vi "Create Log Sink Reference.vi"(8 "Error In":errorcluster, 11 "Log Sink":refnum<class "Log Sink.lvclass">) -> (0 "Error Out":errorcluster, 3 "Log Sink Reference":refnum<data-value>)   [LabVIEW 2016, in "Stream Log.lvlib" / "Log Sink.lvclass"]
doc: "--\nCopyright © 2017 Composed SystemsI All rights reserved.\n\nAuthor: Jon McBee <jon.mcbee@composed.io>\n\nThis library is provided \"AS IS\" ,WITHOUT WARRANTIES OR\nCONDITIONS OF ANY KIND, either express or implied.\n\nComposed Systems -- composed.io\n\nStream 0.0.1.1\nJon McBee - Composed Systems\nCopyright (c) 2017, Composed Systems"
uses:
  <userlib>/Composed Systems/Stream/Log/Log Sink/Log Sink.lvclass
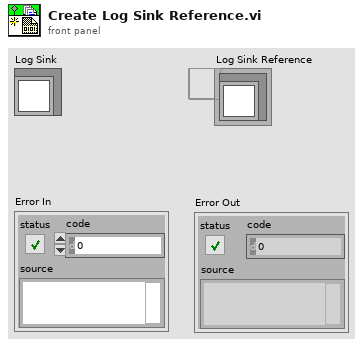
[diagram p1: front panel]
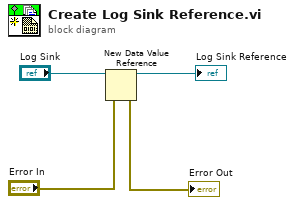
[diagram p0: block diagram]
diagram:
  n1 = New Data Value Reference(data value="Log Sink", error in="Error In") -> (data value reference=→"Log Sink Reference":refnum<data-value>, error out=→"Error Out":errorcluster)
